vi "Hunters Crack Pipes.vi"() -> ()   [LabVIEW 2020]
uses:
  Desktop/tony/Labview Collider/Search Both Address.vi/fc8f06de-4352-3fe5-ca1e-410684fae83f.vi
  Desktop/tony/Labview Collider/Search Both Address.vi/c43f61cc-456e-3fd0-4807-e93e1587c13f.vi
  Desktop/tony/Labview Collider/Search Both Address.vi/fc8f06de-4352-3fe5-ca1e-410684fae83f.vi/d4db2432-cc9c-482c-8957-dac855435ef6.vi
  Desktop/tony/Labview Collider/Search Both Address.vi/fc8f06de-4352-3fe5-ca1e-410684fae83f.vi/86fbf154-bd7b-49a2-8ab2-a837b2a95f24.vi
  Desktop/tony/Labview Collider/Search Both Address.vi/fc8f06de-4352-3fe5-ca1e-410684fae83f.vi/3b95b01e-1ec2-4565-bcd9-7606a5281010.vi
  Desktop/tony/Labview Collider/Search Both Address.vi/fc8f06de-4352-3fe5-ca1e-410684fae83f.vi/96a08935-737a-44b2-979c-a81d56408f7e.vi
  Desktop/tony/Labview Collider/Search Both Address.vi/c43f61cc-456e-3fd0-4807-e93e1587c13f.vi/d4db2432-cc9c-482c-8957-dac855435ef6.vi
  Desktop/tony/Labview Collider/Search Both Address.vi/c43f61cc-456e-3fd0-4807-e93e1587c13f.vi/86fbf154-bd7b-49a2-8ab2-a837b2a95f24.vi
  Desktop/tony/Labview Collider/Search Both Address.vi/c43f61cc-456e-3fd0-4807-e93e1587c13f.vi/3b95b01e-1ec2-4565-bcd9-7606a5281010.vi
  Desktop/tony/Labview Collider/Search Both Address.vi/c43f61cc-456e-3fd0-4807-e93e1587c13f.vi/96a08935-737a-44b2-979c-a81d56408f7e.vi
  Desktop/tony/Labview Collider/Search Both Address.vi/fc8f06de-4352-3fe5-ca1e-410684fae83f.vi/d4db2432-cc9c-482c-8957-dac855435ef6.vi/6eaecd13-6e48-4772-a921-b51ebdf84d88.vi
  Desktop/tony/Labview Collider/Search Both Address.vi/fc8f06de-4352-3fe5-ca1e-410684fae83f.vi/d4db2432-cc9c-482c-8957-dac855435ef6.vi/d2d5f2b7-06f4-47f6-971c-049c3fdbb653.vi
  Desktop/tony/Labview Collider/Search Both Address.vi/fc8f06de-4352-3fe5-ca1e-410684fae83f.vi/3b95b01e-1ec2-4565-bcd9-7606a5281010.vi/6eaecd13-6e48-4772-a921-b51ebdf84d88.vi
  Desktop/tony/Labview Collider/Search Both Address.vi/fc8f06de-4352-3fe5-ca1e-410684fae83f.vi/3b95b01e-1ec2-4565-bcd9-7606a5281010.vi/d2d5f2b7-06f4-47f6-971c-049c3fdbb653.vi
  Desktop/tony/Labview Collider/Search Both Address.vi/fc8f06de-4352-3fe5-ca1e-410684fae83f.vi/96a08935-737a-44b2-979c-a81d56408f7e.vi/6eaecd13-6e48-4772-a921-b51ebdf84d88.vi
  Desktop/tony/Labview Collider/Search Both Address.vi/fc8f06de-4352-3fe5-ca1e-410684fae83f.vi/96a08935-737a-44b2-979c-a81d56408f7e.vi/d2d5f2b7-06f4-47f6-971c-049c3fdbb653.vi
  Desktop/tony/Labview Collider/Search Both Address.vi/c43f61cc-456e-3fd0-4807-e93e1587c13f.vi/d4db2432-cc9c-482c-8957-dac855435ef6.vi/6eaecd13-6e48-4772-a921-b51ebdf84d88.vi
  Desktop/tony/Labview Collider/Search Both Address.vi/c43f61cc-456e-3fd0-4807-e93e1587c13f.vi/d4db2432-cc9c-482c-8957-dac855435ef6.vi/d2d5f2b7-06f4-47f6-971c-049c3fdbb653.vi
  Desktop/tony/Labview Collider/Search Both Address.vi/c43f61cc-456e-3fd0-4807-e93e1587c13f.vi/3b95b01e-1ec2-4565-bcd9-7606a5281010.vi/6eaecd13-6e48-4772-a921-b51ebdf84d88.vi
  Desktop/tony/Labview Collider/Search Both Address.vi/c43f61cc-456e-3fd0-4807-e93e1587c13f.vi/3b95b01e-1ec2-4565-bcd9-7606a5281010.vi/d2d5f2b7-06f4-47f6-971c-049c3fdbb653.vi
  Desktop/tony/Labview Collider/Search Both Address.vi/c43f61cc-456e-3fd0-4807-e93e1587c13f.vi/96a08935-737a-44b2-979c-a81d56408f7e.vi/6eaecd13-6e48-4772-a921-b51ebdf84d88.vi
  Desktop/tony/Labview Collider/Search Both Address.vi/c43f61cc-456e-3fd0-4807-e93e1587c13f.vi/96a08935-737a-44b2-979c-a81d56408f7e.vi/d2d5f2b7-06f4-47f6-971c-049c3fdbb653.vi
  <vilib>/Utility/file.llb/Write Delimited Spreadsheet.vi
  <vilib>/Utility/file.llb/Write Delimited Spreadsheet (string).vi
  <vilib>/Comparison/Less/Less Functor/Less Functor.lvclass
panel:
  out "output cluster":cluster{dbl, "data":string}
  out "Time Has Elapsed":bool
  in  "Reset Button":bool
  in  "Auto Reset":bool
  in  "Tab Control":enum32{"Main", "Samples"}(tab)
  in  "Stop":bool
  out "Elapsed Time":string caption="Elapsed Time Text"
  in  "?":bool
  out "Key":string
  out "Add U":string
  out "Add C":string
  out "?":dbl(graph)
  out "Attempts Addresses":string
  in  "Throttle":u32
  out "Key's /s":dbl format="%#.0f"
  out "Sms Sent":bool
  in  "Text Enable":bool
  out "Found":bool
  in  "Threads":i32(ring)=1 items=["Threads", "1", "2", "3", "4", "5", "6", "7", "8", "9", "10", "11", "12", "13", "14", "15", "16", "17", "18", "19", "20", "21", "22", "23", "24", "25", "26", "27", "28", "29", "30", "31", "32", "33", "34", "35", "36", "37", "38", "39", "40", "41", "42", "43", "44", "45", "46", "47", "48", "49", "50", "51", "52", "53", "54", "55", "56", "57", "58", "59", "60", "61", "62", "63", "64", "65", "66", "67", "68", "69", "70", "71", "72", "73", "74", "75", "76", "77", "78", "79", "80"]
  in  "Select Address File    -------------------------------------------->":path
  out "Addrs  /Sec":dbl format="%#.0f"
  in  "?":bool
  out "?":string
  in  "?":bool
  in  "?":u16(ring) items=["Settings", "Configure"]
  out "File Count":string
  in  "?":bool
  in  "Apend To File?":bool
  in  "?":bool
  out "Samples":string[][](table)
  in  "?":bool
  in  "# Samples":i32
  out "?":i32
  in  "Select  Saved Samples File":path
  # "Hunter's Crack Pipe"
  # "Keys Sec"
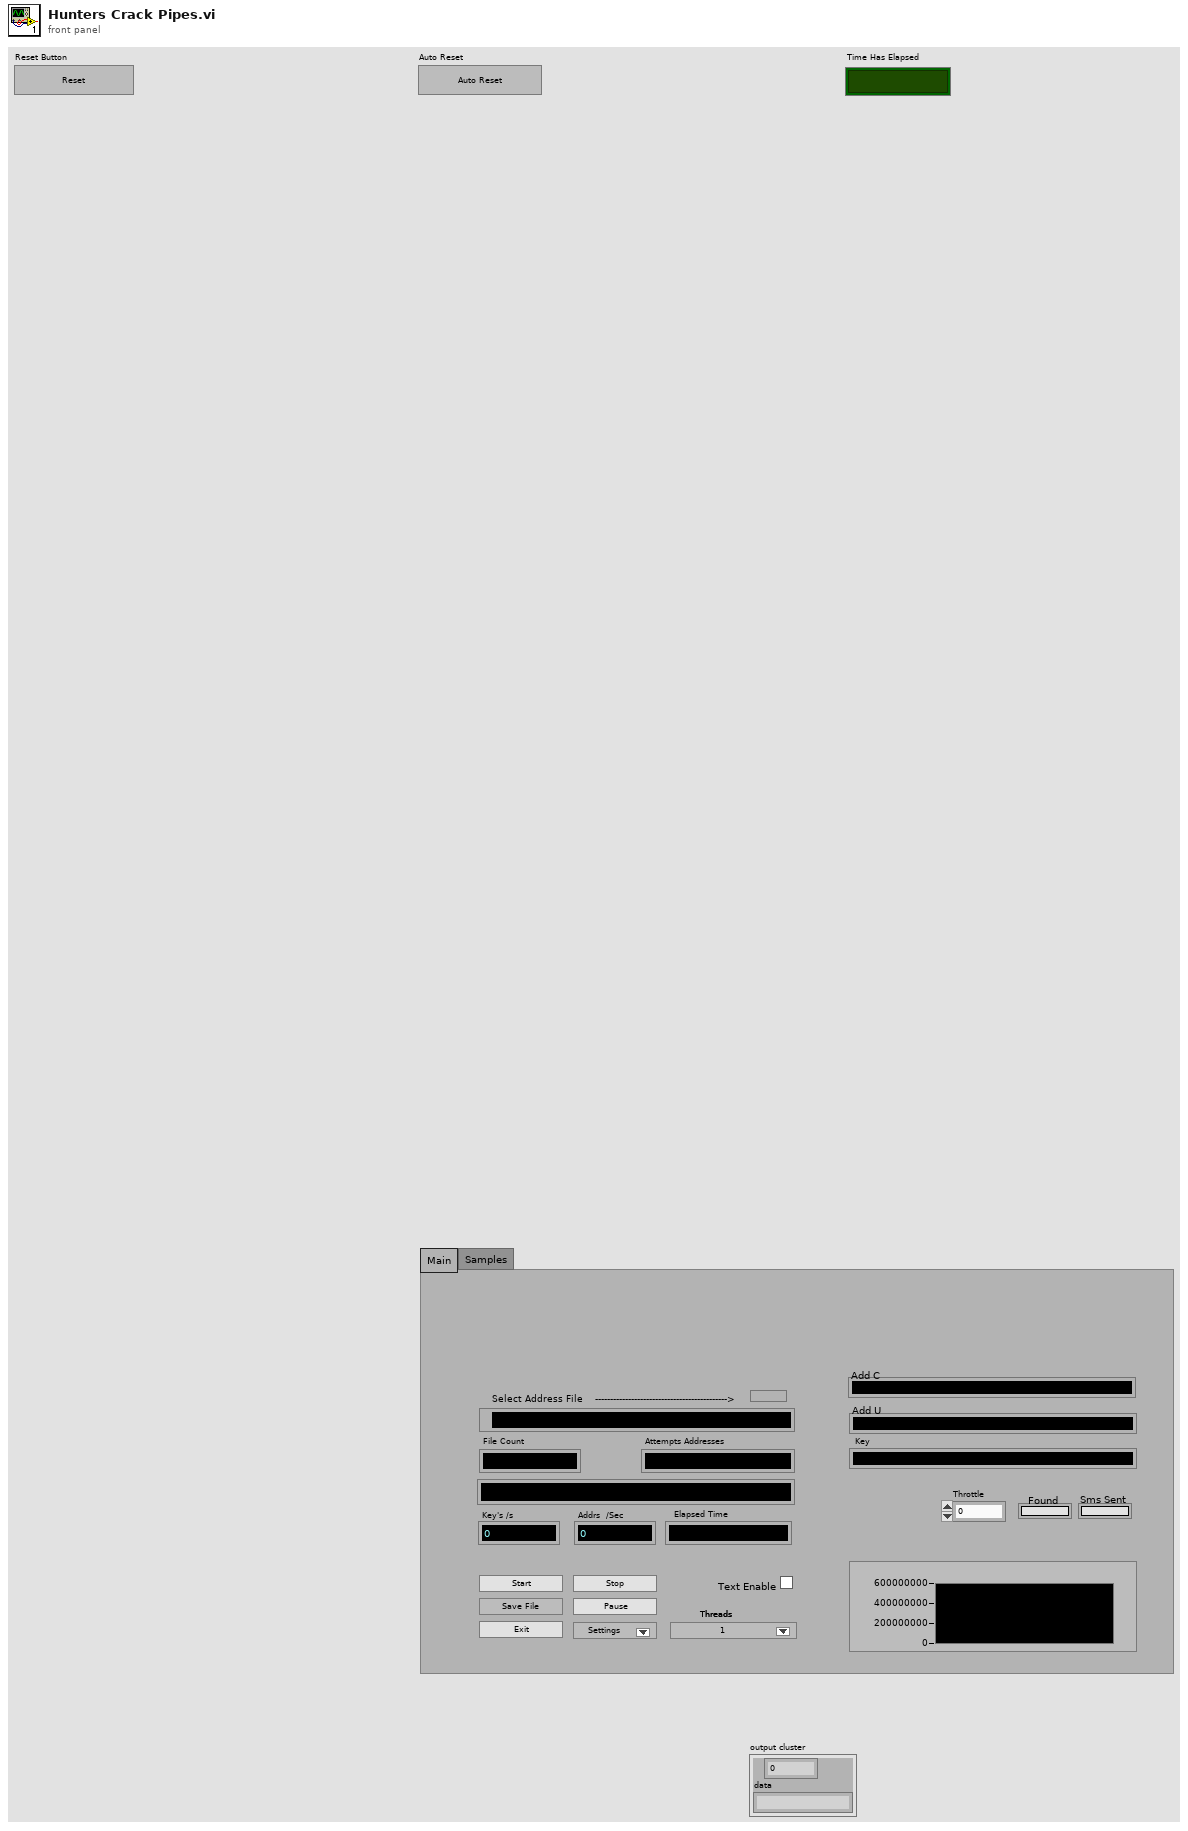
[diagram p1: front panel]
types:
  T1 = enum8{"Enabled", "Disabled", "Disabled and Grayed Out"}
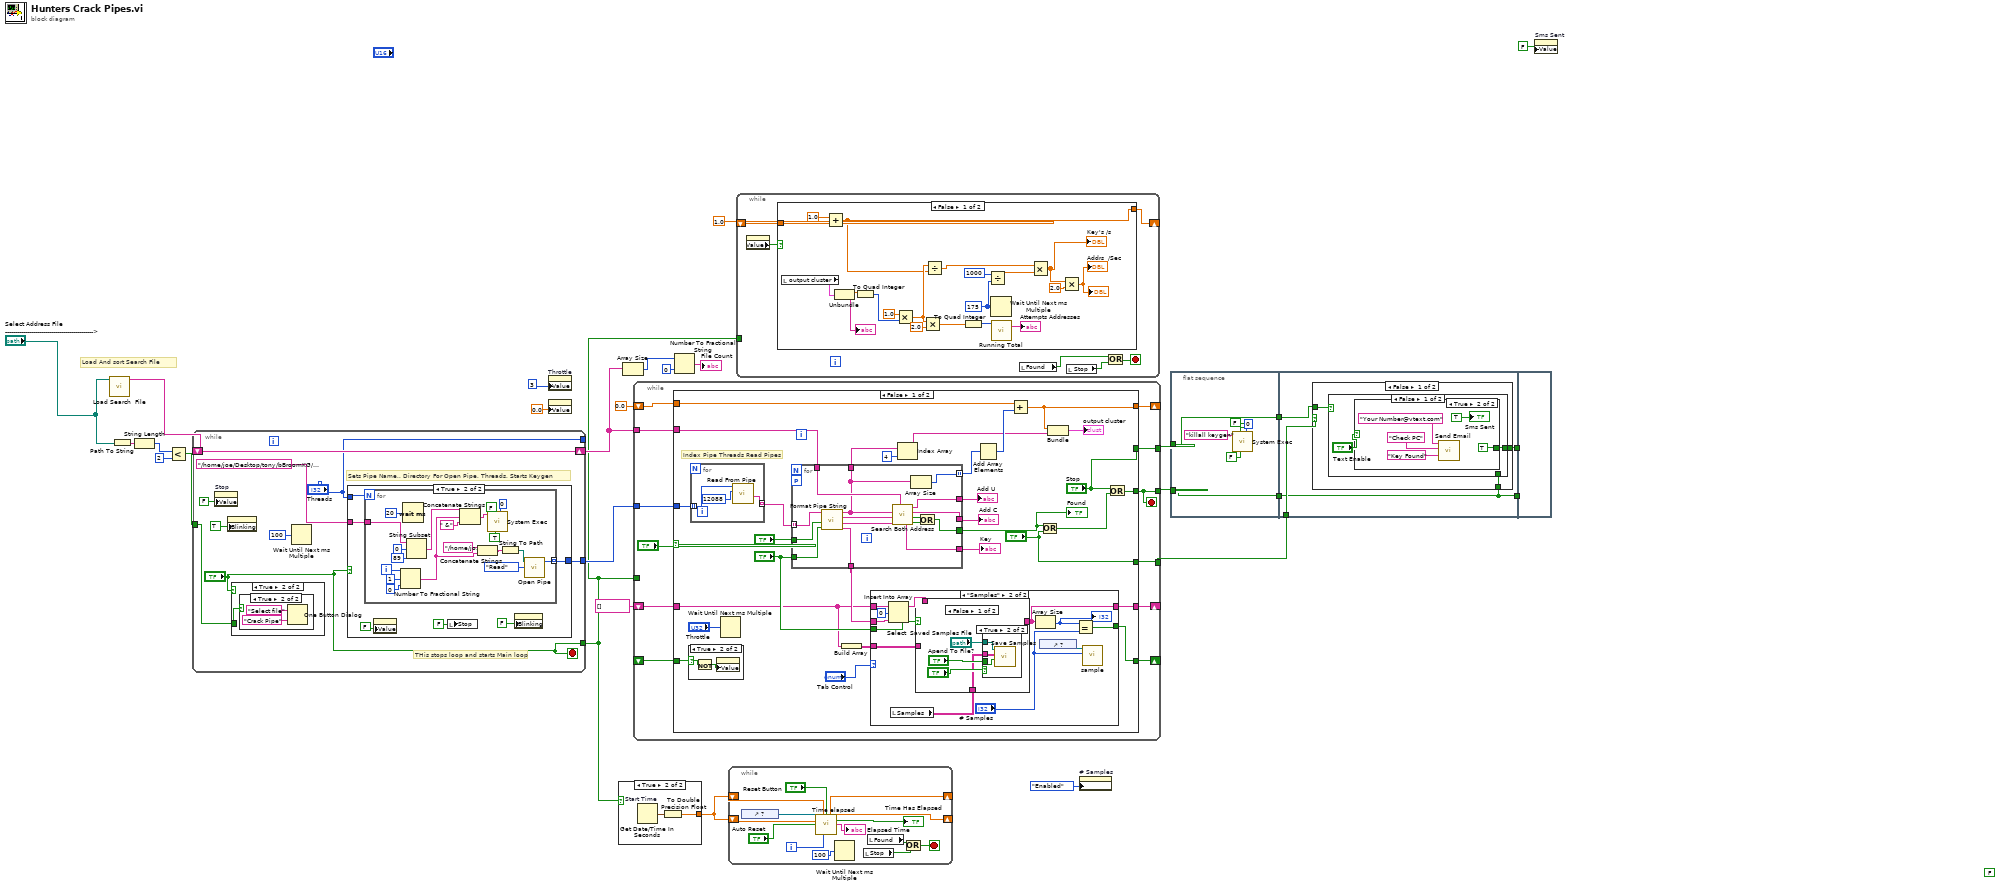
[diagram p0: block diagram]
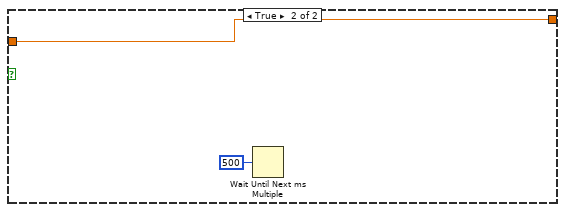
[diagram p3: hidden frame]
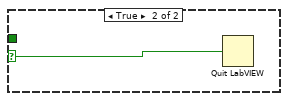
[diagram p9: hidden frame]
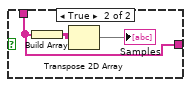
[diagram p12: hidden frame]
diagram:
  (unwired) FALSE
  # "Load And sort Search File"
  n1 = call "Load Search  File.vi"("Select Address File           --------------------------->"="Select Address File    -------------------------------------------->") -> ("sorted array"=w19:string[])  [unwired: 10 in]
  n2 = Path To String(path="Select Address File    -------------------------------------------->") -> (string=w18:string)
  n3 = String Length(string=w18) -> (length=w17:i32)
  n4 = Less?(x=w17, y=2) -> (x < y?=w15:bool)
  n5 = while {
    tunnel: [w36] -> w10
    tunnel: ["Threads"] -> _
    shift-right: [w34] -> w6
    shift-left: w19 -> [w34]
    tunnel: ["?"] -> w2
    tunnel: w15 -> [w33]
    stop <- "?" stop-if-true
    # "THis stops loop and starts Main loop"
    # "Sets Pipe Name,, Directory For Open Pipe, Threads, Starts Keygen"
    n6 = property on="Stop" class="Bool (strict)"("Value"=FALSE ("Stop")) -> ()  [unwired: 2 in, 2 out]
    n7 = property class="Bool (strict)"("Blinking"=TRUE) -> ()  [unwired: 2 in, 2 out]
    n8 = case shown="True" "?" {
      tunnel: w33 -> [_ w37]
      frame False {
      }
      frame True {
        n9 = case shown="True" w37 {
          frame False {
          }
          frame True {
            n10 = One Button Dialog(message="Select file", button name ("OK")="Crack Pipe") -> ()  [unwired: 1 out]
          }
        }
      }
    }
    n11 = Wait Until Next ms Multiple(millisecond multiple=u32 100) -> ()  [unwired: 1 out]
    n12 = case shown="True" "?" {
      tunnel: [_ w43] -> w36
      tunnel: "Threads" -> [_ w44]
      tunnel: "/home/joe/Desktop/tony/bBroomKG/keygen > /home/joe/Desktop/tony/bBroomKG/hunterscrackpipe0" ("command line") -> [_ w40]
      frame False {
      }
      frame True {
        n13 = for {
          N: w44 -> [_]
          tunnel: [w50] -> w43 mode=indexing
          tunnel: w40 -> [w47]
          i -> [w55]
          n14 = Number To Fractional String(number=w55, width (-)=i16 1, precision (6)=i16 0) -> (F-format string=w54:string)  [unwired: 1 in]
          n15 = Wait (ms)(milliseconds to wait=u32 20) -> ()  [unwired: 1 out]
          n16 = String Subset(string=w47, offset (0)=0, length (rest)=89 ("length (rest)")) -> (substring=w62:string)
          n17 = Concatenate Strings(w62, w54, " &" ("string")) -> (w48:string)
          n18 = Concatenate Strings("/home/joe/Desktop/tony/bBroomKG/hunterscrackpipe", w54) -> (w49:string)
          n19 = call <vilib>:"System Exec.vi"("expected output size  (4096)"=u32 0, "run minimized? (F)"=TRUE, "wait until completion? (T)"=FALSE, "command line"=w48) -> ()  [unwired: 4 in, 4 out]
          n20 = String To Path(string=w49) -> (path=w51:path)
          n21 = call <vilib>:"Open Pipe.vi"("mode"=enum8{"Read", "Write"}."Read", "path to named pipe"=w51) -> ("file descriptor"=w50:i32)  [unwired: 2 in, 1 out]
        }
        n22 = property class="Bool (strict)"("Value"=FALSE ("Start Collider")) -> ()  [unwired: 2 in, 2 out]
        n23 = local write "Stop"(FALSE ("Stop")) -> ()
        n24 = property class="Bool (strict)"("Blinking"=FALSE) -> ()  [unwired: 2 in, 2 out]
      }
    }
  }
  n25 = property on="Throttle" class="DigNum (strict)"("Value"=u32 3 ("Throttle")) -> ()  [unwired: 2 in, 2 out]
  n26 = property class="WFChart (strict)"("Value"=0.0) -> ()  [unwired: 2 in, 2 out]
  n27 = case shown="True" w2 {
    tunnel: [_ w65] -> w5
    frame False {
    }
    frame True {
      n28 = Get Date/Time In Seconds "Start Time"() -> (seconds since 1Jan1904=w66:timestamp)
      n29 = To Double Precision Float(number=w66) -> (double precision float=w65:dbl)
    }
  }
  n30 = Array Size(array=w6) -> (size(s)=w21:i32)
  n31 = while {
    tunnel: w10 -> [w78]
    tunnel: [w75] -> w9
    tunnel: [w68] -> w22
    tunnel: w2 -> [_]
    shift-right: [w76] -> _
    shift-left: 0.0 -> [w77]
    shift-right: [w71] -> _
    shift-left: string[] [] ("sorted array") -> [w74]
    shift-right: [w73] -> _
    shift-left: _ -> [w72]
    tunnel: w6 -> [w70]
    tunnel: [w67] -> w4
    stop <- w68 stop-if-true
    n32 = case shown="False" "?" {
      tunnel: w78 -> [w89 _]
      tunnel: [w99 _] -> w68
      tunnel: w77 -> [w107 w151]
      tunnel: [w91 w151] -> w76
      tunnel: ["?" _] -> w75
      tunnel: w74 -> [w80 _]
      tunnel: [w105 _] -> w73
      tunnel: w72 -> [w104 _]
      tunnel: [w103 _] -> w71
      tunnel: w70 -> [w88 _]
      tunnel: ["Stop" _] -> w67
      frame False {
        # "Index Pipe Threads Read Pipes"
        n33 = case shown="True" w104 {
          selector: w104 -> [_ w150]
          frame False {
          }
          frame True {
            n34 = Not(x=w150) -> (.not. x?=w149:bool)
            n35 = property class="Bool (strict)"("Value"=w149) -> ()  [unwired: 2 in, 2 out]
          }
        }
        n36 = for {
          tunnel: w89 -> [w125] mode=indexing
          tunnel: [w123] -> w85 mode=indexing
          n37 = call <vilib>:"Read From Pipe.vi"("file descriptor"=w125, "bytes to read"=12088) -> ("data"=w123:string)  [unwired: 2 in, 4 out]
        }
        n38 = Wait Until Next ms Multiple(millisecond multiple="Throttle") -> ()  [unwired: 1 out]
        n39 = for {
          tunnel: w85 -> [w114] mode=indexing
          tunnel: w88 -> [w122]
          workers-P: _ -> [_]
          tunnel: [w121] -> w93
          tunnel: [w110] -> w96
          tunnel: [w120] -> w95
          tunnel: [w119] -> w94
          tunnel: [w113] -> w97
          tunnel: "?" -> [w112]
          tunnel: "?" -> [w111]
          tunnel: [w109] -> w90 mode=indexing
          tunnel: [w108] -> w83
          n40 = call "Format Pipe String.vi"("Grab samples"=w111, "Write File"=w112, "data"=w114) -> ("Samples"=w113:string, "Key"=w115:string[], "Address C"=w116:string[], "Address U"=w108:string[])  [unwired: 4 in, 1 out]
          n41 = call "Search Both Address.vi"("Address U"=w108, "Address C"=w116, "Key"=w115, "sorted array"=w122) -> ("Key  U"=w119:string, "Address U"=w110:string, "Address C"=w120:string, "Match U"=w118:bool, "Match C"=w117:bool)  [unwired: 2 in]
          n42 = Array Size(array=w108) -> (size(s)=w109:i32)
          n43 = Or(x=w118, y=w117) -> (x .or. y?=w121:bool)
        }
        "Found" <- w93
        "Add C" <- w95
        "Add U" <- w96
        "Key" <- w94
        n44 = Build Array(w80) -> (w79:string[][])
        n45 = case shown="\"Samples\"" "Tab Control" {
          tunnel: w80 -> [w126 w138]
          tunnel: [_ w137] -> w105
          tunnel: "?" -> [_ w135]
          tunnel: w97 -> [_ w134]
          tunnel: [w126 w133] -> w103
          tunnel: w79 -> [_ w128]
          frame "Main", Default {
          }
          frame "Samples" {
            n46 = Insert Into Array(array=w138, index=0, new element=w134) -> (w136:string[])
            n47 = local read "Samples"() -> (w127:string[][])
            n48 = case shown="False" w135 {
              tunnel: w136 -> [_ w146]
              tunnel: [_ w146] -> w133
              tunnel: w128 -> [_ _]
              tunnel: w127 -> [w139 _]
              frame False {
                n49 = case shown="True" "?" {
                  tunnel: "Apend To File?" -> [_ w145]
                  tunnel: "Select  Saved Samples File" -> [_ w144]
                  tunnel: w139 -> [_ w143]
                  frame False {
                  }
                  frame True {
                    n50 = call "Save Samples.vi"("Boolean"=w145, "transposed array"=w143, "Select  Saved Samples File"=w144) -> ()  [unwired: 9 in]
                  }
                }
              }
              frame True {
                n51 = Build Array(w146) -> (w148:string[][])
                n52 = Transpose 2D Array(2D array=w148) -> (transposed array=→"Samples":string[][])
              }
            }
            n53 = Array Size(array=w133) -> (size(s)=w131:i32)
            "?" <- w131
            n54 = control-ref of="?"() -> (w130:refnum<vi>)
            n55 = Equal?(x=w131, y="# Samples") -> (x = y?=w137:bool)
            n56 = call "sample.vi"("# Samples"="# Samples", "Boolean in"=w130) -> ()  [unwired: 10 in]
          }
        }
        n57 = Index Array(array=w83, index=4) -> (element=w81:string)
        n58 = Add Array Elements(numeric array=w90) -> (sum=w87:i32)
        n59 = Add(x=w107, y=w87) -> (x+y=w91:dbl)
        n60 = Or(x=w93, y="?") -> (x .or. y?=w100:bool)
        n61 = Bundle(w91, "standard output"=w81) -> (→"output cluster":cluster{dbl, "standard output":string})  [unwired: 1 in]
        n62 = Or(x="Stop", y=w100) -> (x .or. y?=w99:bool)
      }
      frame True {
      }
    }
  }
  n63 = Number To Fractional String(number=w21, precision (6)=i16 0) -> (F-format string=→"File Count":string)  [unwired: 2 in]
  n64 = while {
    shift-right: [w161] -> _
    shift-left: w5 -> [w165]
    shift-right: [w162] -> _
    shift-left: w5 -> [w164]
    i -> [w157]
    stop <- w153 stop-if-true
    n65 = control-ref of="?"() -> (w156:refnum<vi>)
    n66 = call "Time elapsed.vi"("Boolean in"=w156, "Numeric 3"=w164, "Reset Button"="Reset Button", "Numeric 4"=w165, "Auto Reset"="Auto Reset", "Numeric in"=w157) -> ("Present (s) 2"=w162:dbl, "Present (s)"=w161:dbl, "Time has Elapsed"=→"Time Has Elapsed":bool, "Elapsed Time Text"=→"Elapsed Time":string)  [unwired: 4 in, 2 out]
    n67 = Wait Until Next ms Multiple(millisecond multiple=u32 100) -> ()  [unwired: 1 out]
    n68 = local read "Stop"() -> (w154:bool)
    n69 = local read "Found"() -> (w155:bool)
    n70 = Or(x=w155, y=w154) -> (x .or. y?=w153:bool)
  }
  n71 = while {
    shift-right: [w170] -> _
    shift-left: 1.0 -> [w171]
    tunnel: w2 -> [_]
    stop <- w166 stop-if-true
    n72 = property class="Bool (strict)"() -> ("Value"=w167:bool)  [unwired: 2 in, 2 out]
    n73 = case shown="False" w167 {
      tunnel: w171 -> [w183 w193]
      tunnel: [w181 w193] -> w170
      frame False {
        w184 = u32 175 ("millisecond multiple")
        n74 = local read "output cluster"() -> (w173:cluster{dbl, "data":string})
        n75 = Add(x=1.0, y=w183) -> (x+y=w181:dbl)
        n76 = Unbundle(w173) -> (w174:dbl, "data"=→"?":string)
        n77 = To Quad Integer(1:w174) -> (0:w175:i64)
        n78 = Multiply(x=1.0, y=w175) -> (x*y=w189:dbl)
        n79 = Multiply(x=w189, y=2.0 ("x")) -> (x*y=w188:dbl)
        n80 = Divide(x=w189, y=w181) -> (x/y=w190:dbl)
        n81 = To Quad Integer(1:w188) -> (0:w187:i64)
        n82 = Divide(x=u32 1000 ("y"), y=w184) -> (x/y=w186:dbl)
        n83 = Wait Until Next ms Multiple(millisecond multiple=w184) -> ()  [unwired: 1 out]
        n84 = call "Running Total.vi"("Numeric 4"=w187) -> ("String"=→"Attempts Addresses":string)  [unwired: 10 in]
        n85 = Multiply(x=w190, y=w186) -> (x*y=w177:dbl)
        "Key's /s" <- w177
        n86 = Multiply(x=w177, y=2.0) -> (x*y=→"Addrs  /Sec" →"?":dbl)
      }
      frame True {
        n87 = Wait Until Next ms Multiple(millisecond multiple=u32 500) -> ()  [unwired: 1 out]
      }
    }
    n88 = local read "Found"() -> (w169:bool)
    n89 = local read "Stop"() -> (w168:bool)
    n90 = Or(x=w169, y=w168) -> (x .or. y?=w166:bool)
  }
  n91 = property on="# Samples" class="DigNum (strict)"("DisabledEnum"=T1."Enabled" ("Disabled")) -> ()  [unwired: 2 in, 2 out]
  n92 = flat-sequence {
    tunnel: w22 -> [w199]
    tunnel: [w199] -> w26
    tunnel: [w194] -> w25
    tunnel: w4 -> [w194]
    tunnel: w9 -> [w203]
    tunnel: [w202] -> w24
    tunnel: w26 -> [w201]
    tunnel: [w201] -> w23
    tunnel: w25 -> [w200]
    tunnel: w24 -> [_]
    tunnel: w23 -> [_]
    frame #0 {
      n93 = call <vilib>:"System Exec.vi"("expected output size  (4096)"=u32 0, "run minimized? (F)"=FALSE, "wait until completion? (T)"=FALSE, "command line"="killall keygen") -> ()  [unwired: 4 in, 4 out]
    }
    frame #1 {
      n94 = case shown="False" w203 {
        selector: w203 -> [_ w215]
        tunnel: [w206 _] -> w202
        tunnel: w201 -> [w205 _]
        tunnel: w200 -> [w204 _]
        frame False {
          n95 = case shown="False" w204 {
            tunnel: [w208 w214] -> w206
            tunnel: w205 -> [_ w214]
            frame False {
              n96 = case shown="True" "Text Enable" {
                tunnel: [_ TRUE] -> w208
                frame False {
                }
                frame True {
                  n97 = call "Send Email"("Message"="Key Found", "Subject"="Check PC", "Recipients"="Your Number@vtext.com") -> ()  [unwired: 8 in, 1 out]
                  "Sms Sent" <- TRUE ("Sms Sent")
                }
              }
            }
            frame True {
            }
          }
        }
        frame True {
          n98 = Quit LabVIEW(quit? (T)=w215) -> ()
        }
      }
    }
    frame #2 {
    }
  }
  n99 = property on="Sms Sent" class="Bool (strict)"("Value"=FALSE ("Sms Sent")) -> ()  [unwired: 2 in, 2 out]
